vi "Close.vi"(8 "error in (no error)":errorcluster, 11 "NetworkStreamWriter in":refnum<class "Logger.lvclass">) -> (0 "error out":errorcluster)   [LabVIEW 2011, in "Logger.lvclass"]
doc: "This VI closes references internal to the NetworkStreamWriter object. This allows memory to be cleaned up effectively."
uses:
  Logger.lvclass
  Logger.lvclass/Logger.ctl
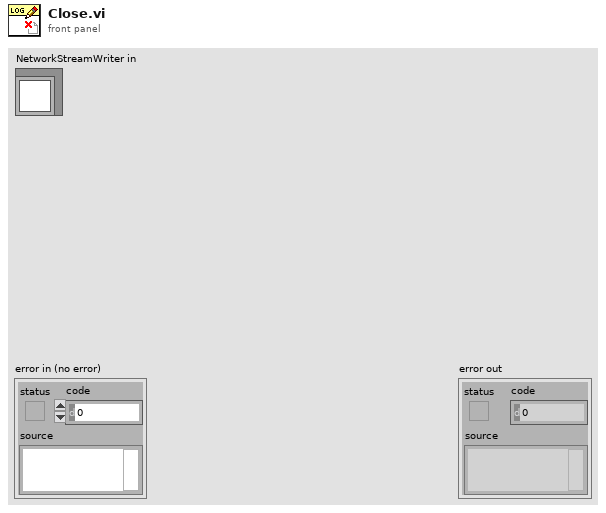
[diagram p1: front panel]
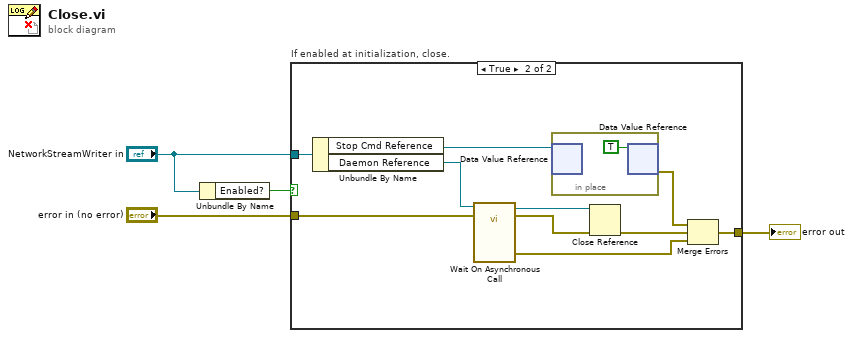
[diagram p0: block diagram]
diagram:
  n1 = Unbundle By Name("NetworkStreamWriter in") -> ("Enabled?"=w1:bool)
  n2 = case "If enabled at initialization, close." shown="True" w1 {
    tunnel: "NetworkStreamWriter in" -> [_ w15]
    tunnel: [w5 w11] -> w4
    tunnel: "error in (no error)" -> [w5 w8]
    frame False {
    }
    frame True {
      n3 = Unbundle By Name(w15) -> ("Stop Cmd Reference"=w14:refnum<data-value>, "Daemon Reference"=w10:refnum<vi>)
      n4 = call-by-ref "Wait On Asynchronous Call"(reference=w10, error in=w8) -> (reference out=w9:refnum<vi>, error out=w7:errorcluster, 0:"error out"=w6:errorcluster)  [unwired: 11 in]
      n5 = in-place {
        n6 = in-place-dvr #1(w14) -> ()  [unwired: 2 out]
        n7 = in-place-dvr #1(TRUE ("data value")) -> (w12:errorcluster)  [unwired: 1 out]
      }
      n8 = Close Reference(reference=w9, error in (no error)=w7) -> (error out=w13:errorcluster)
      n9 = Merge Errors(w12, w13, w6) -> (w11:errorcluster)
    }
  }
  "error out" <- w4
